vi "CAP.vi"(0 "Freq Hz K; M Hz":dbl, 1 "Surface Area 1 NS":dbl, 2 "Permitivity of Free Space":dbl, 3 "er":dbl, 4 "No of NS Pairs on Chip":dbl, 6 "Frequency":dbl, 7 "Gap B/w NS":dbl, 9 "Voltage":dbl) -> (10 "Impedance":dbl, 11 "Power":dbl, 12 "Chip Impedance":dbl, 13 "Chip Power":dbl, 14 "Capacitance of 1 Pair NS":dbl, 15 "Capacitance of 1 Pair":dbl(graph), 16 "Chip Capacitance":dbl, 17 "Chip Energy":dbl, 18 "Energy":dbl)   [LabVIEW 2020]
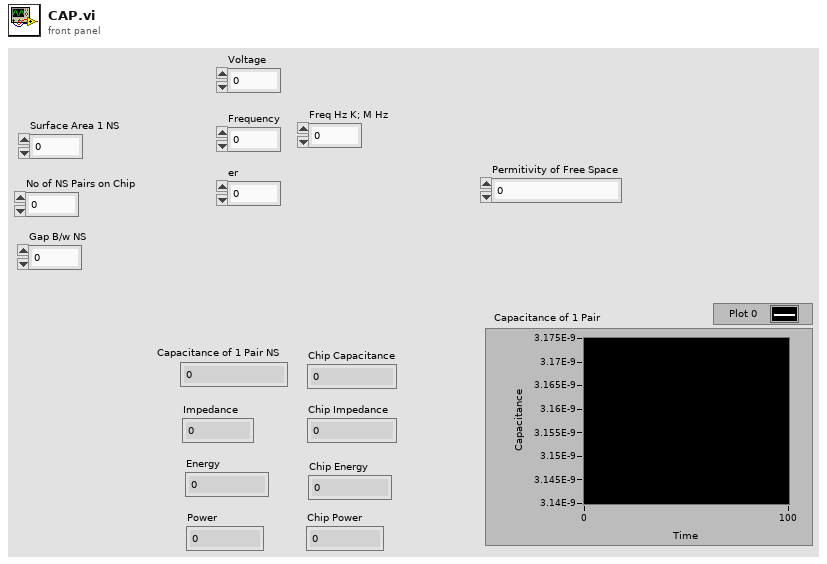
[diagram p1: front panel]
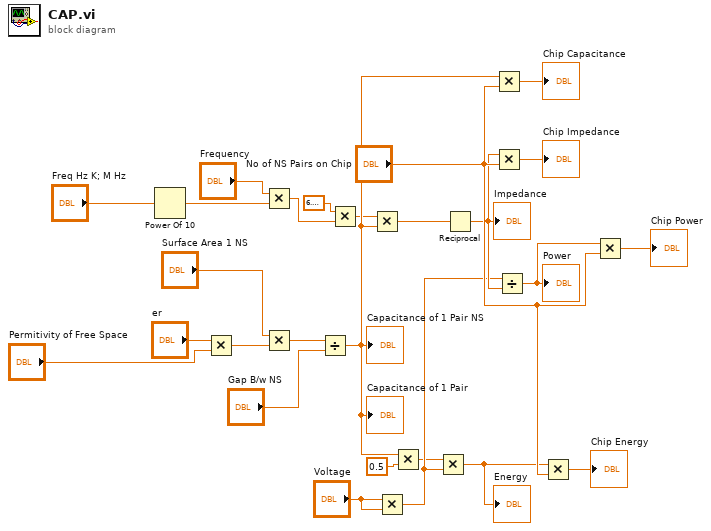
[diagram p0: block diagram]
diagram:
  n1 = Power Of 10(x="Freq Hz K; M Hz") -> (10^x=w12:dbl)
  n2 = Multiply(x="er", y="Permitivity of Free Space") -> (x*y=w2:dbl)
  n3 = Multiply(x="Frequency", y=w12) -> (x*y=w14:dbl)
  n4 = Multiply(x="Surface Area 1 NS", y=w2) -> (x*y=w3:dbl)
  n5 = Divide(x=w3, y="Gap B/w NS") -> (x/y=w20:dbl)
  "Capacitance of 1 Pair NS" <- w20
  "Capacitance of 1 Pair" <- w20
  n6 = Multiply(x=6.283185307179586, y=w14) -> (x*y=w7:dbl)
  n7 = Multiply(x=w7, y=w20) -> (x*y=w8:dbl)
  n8 = Multiply(x="Voltage", y="Voltage") -> (x*y=w10:dbl)
  n9 = Multiply(x=w20, y=0.5) -> (x*y=w6:dbl)
  n10 = Multiply(x=w6, y=w10) -> (x*y=w19:dbl)
  "Energy" <- w19
  n11 = Reciprocal(x=w8) -> (1/x=w22:dbl)
  "Impedance" <- w22
  n12 = Multiply(x=w20, y="No of NS Pairs on Chip") -> (x*y=→"Chip Capacitance":dbl)
  n13 = Multiply(x=w22, y="No of NS Pairs on Chip") -> (x*y=→"Chip Impedance":dbl)
  n14 = Divide(x=w10, y=w22) -> (x/y=w18:dbl)
  "Power" <- w18
  n15 = Multiply(x=w19, y="No of NS Pairs on Chip") -> (x*y=→"Chip Energy":dbl)
  n16 = Multiply(x=w18, y="No of NS Pairs on Chip") -> (x*y=→"Chip Power":dbl)
